vi "PCP SIC Command Answer Q.vi"(11 "error in (no error)":errorcluster) -> (8 "PCP Ans Q":refnum<queue>, 10 "PCP Ans Not":refnum<notifier>, 15 "error out":errorcluster)   [LabVIEW 2011]
uses:
  PCP Command Return.ctl
  PCP Commands.ctl
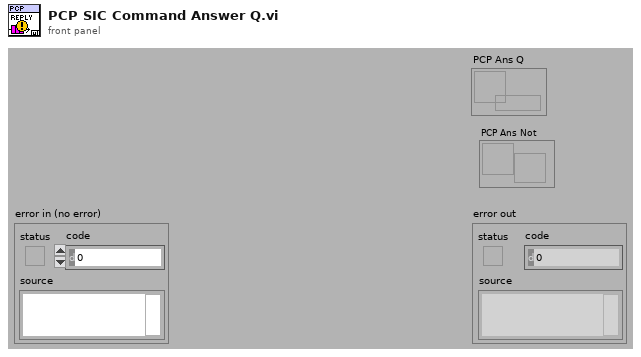
[diagram p1: front panel]
types:
  T1 = typedef "PCP Command Return.ctl" = cluster{"Action":T2, "Data in return":variant}
  T2 = typedef "PCP Commands.ctl" = enum16{"do not use HE - Help", "RDd - Most used inputs", "RA - All analog inputs", "RE n Reset DO n", "SE n Set DO n", "RP - Get digital inputs", "VA d Set AO A  Motor Volt", "VB d Set AO B  Cable Resistance", "VEr - Get Version", "DYp - Depth counter", "DR - Reset Depth Counter", "DS n Set Depth options(0-3)", "do not use ME - Manual mode enabled", "MD - Manual mode disabled", "ID - Get ID(2001)", "TS - Get Timestamp", "TO d(s)  Set timeout", "do not use LO n Start Loop Mode(1,2)", "AL n RD&LO variation", "ST - Stop Loop Mode"}
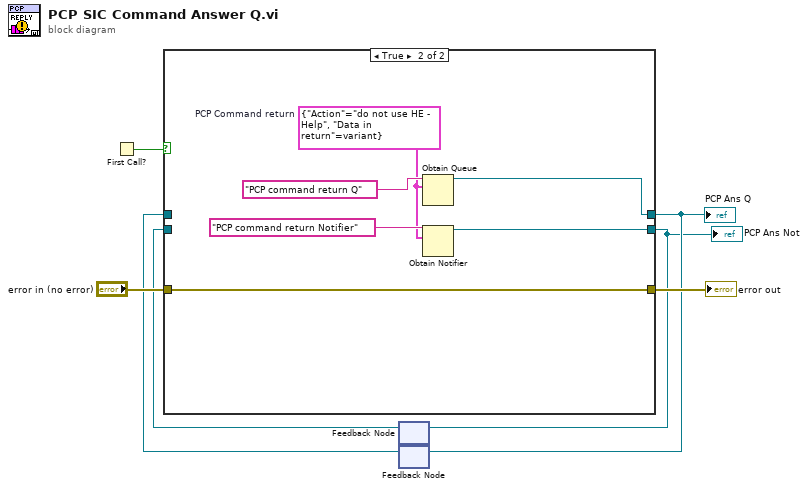
[diagram p0: block diagram]
diagram:
  n1 = First Call?() -> (First Call?: T/F=w5:bool)
  n2 = feedback #1() -> (w1:refnum<notifier>)  [unwired: 1 in]
  n3 = feedback #2() -> (w3:refnum<queue>)  [unwired: 1 in]
  n4 = case shown="True" w5 {
    tunnel: [w10 w16] -> w7
    tunnel: "error in (no error)" -> [w10 w16]
    tunnel: [w9 w14] -> w4
    tunnel: w3 -> [w9 _]
    tunnel: [w8 w11] -> w2
    tunnel: w1 -> [w8 _]
    frame False {
    }
    frame True {
      w12 = T1 {"Action"=enum."do not use HE - Help", "Data in return"=variant}  # PCP Command return
      n5 = Obtain Queue(name (unnamed)="PCP command return Q", element data type=w12) -> (queue out=w14:refnum<queue>)  [unwired: 3 in, 2 out]
      n6 = Obtain Notifier(name (unnamed)="PCP command return Notifier", notification data type=w12) -> (notifier out=w11:refnum<notifier>)  [unwired: 2 in, 2 out]
    }
  }
  "error out" <- w7
  "PCP Ans Q" <- w4
  "PCP Ans Not" <- w2
  n7 = feedback-in #1(w2) -> ()
  n8 = feedback-in #2(w4) -> ()
